vi "create raster.vi"(11 "Array [x start, x length]":cluster{"x start":i32, "x length":i32}[](array[cluster])) -> (2 "raster image":bool[][](array[boolean]))   [LabVIEW 2009]
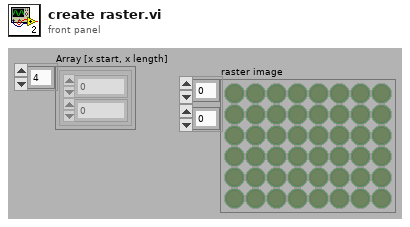
[diagram p1: front panel]
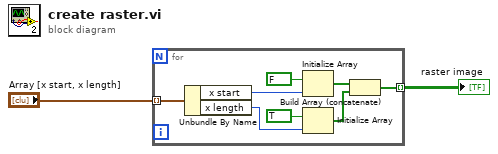
[diagram p0: block diagram]
diagram:
  n1 = for {
    tunnel: "Array [x start, x length]" -> [w9] mode=indexing
    tunnel: [w3] -> w1 mode=indexing
    n2 = Unbundle By Name(w9) -> ("x start"=w6:i32, "x length"=w8:i32)
    n3 = Initialize Array(FALSE, w6) -> (w5:bool[])
    n4 = Initialize Array(TRUE, w8) -> (w4:bool[])
    n5 = Build Array (concatenate)(w5, w4) -> (w3:bool[])
  }
  "raster image" <- w1
